vi "Attach Params.vi"(8 "Error in":errorcluster caption="Error in (no error)", 10 "URL":string, 11 "Param array":T1[](array[typedef])) -> (0 "Error out":errorcluster, 2 "URL with params":string)   [LabVIEW 2018]
uses:
  TypeDef/Param.ctl
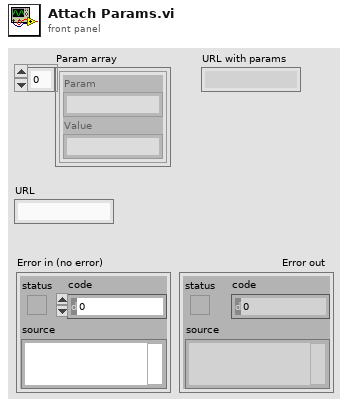
[diagram p1: front panel]
types:
  T1 = typedef "Param.ctl" = cluster{"Param":string, "Value":string}
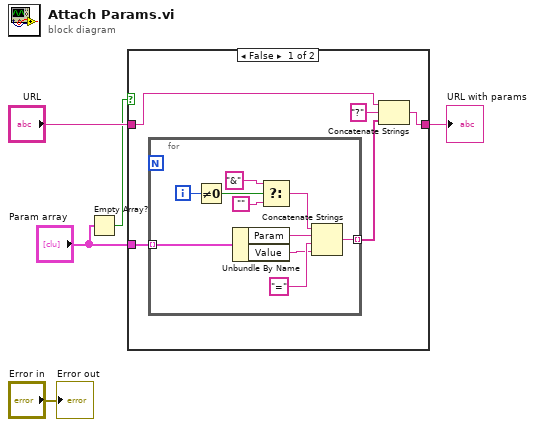
[diagram p0: block diagram]
diagram:
  n1 = Empty Array?(array="Param array") -> (empty?=w3:bool)
  n2 = case shown="False" w3 {
    tunnel: "Param array" -> [w10 _]
    tunnel: "URL" -> [w9 w21]
    tunnel: [w8 w21] -> w5
    frame False {
      n3 = for {
        tunnel: w10 -> [w20] mode=indexing
        tunnel: [w16] -> w6 mode=indexing
        i -> [w15]
        n4 = Not Equal To 0?(x=w15) -> (x != 0?=w14:bool)
        n5 = Unbundle By Name(w20) -> ("Param"=w19:string, "Value"=w17:string)
        n6 = Select(t="&" ("string"), s=w14, f="") -> (s? t:f=w12:string)
        n7 = Concatenate Strings(w12, w19, "=" ("string"), w17) -> (w16:string)
      }
      n8 = Concatenate Strings(w9, "?" ("string"), w6) -> (w8:string)
    }
    frame True {
      # "No Params to attach"
    }
  }
  "URL with params" <- w5
  "Error out" <- "Error in"
